vi "Launcher - Graph Master.vi"(6 "Worker Alias":string="Graph Master", 8 "error in":errorcluster, 9 "Initialization Data":T1, 11 "Graph Master in":refnum<class "Graph Master.lvclass">) -> (0 "error out":errorcluster)   [LabVIEW 2023, in "Graph Master.lvclass"]
doc: "This VI launches the Head Worker of a Workers application."
uses:
  Graph Master.lvclass
  Initialization Data.ctl
  Response Cases.ctl
  C:/Program Files/National Instruments/LabVIEW 2023/vi.lib/addons/_Workers/Library/Classes/Worker/Worker.lvclass
  Graph Master.lvclass/Graph Master.ctl
  <vilib>/addons/_Workers/Debugger/Debug Client/Debug Client.lvlib
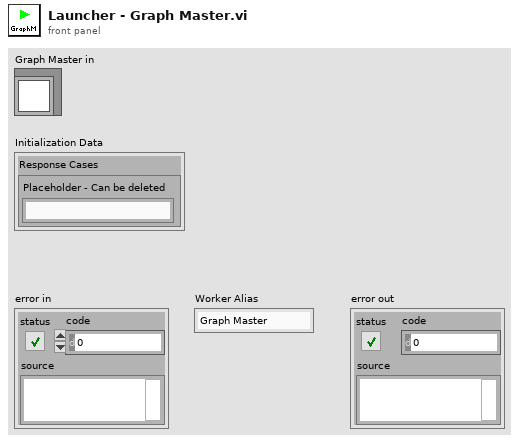
[diagram p1: front panel]
types:
  T1 = typedef "Graph Master.lvclass/Initialization Data.ctl" = cluster{"Response Cases":T2}
  T2 = typedef "Graph Master.lvclass/Response Cases.ctl" = cluster{"Placeholder - Can be deleted":string}
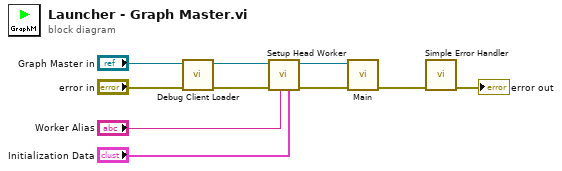
[diagram p0: block diagram]
diagram:
  n1 = call <vilib>:"Debug Client Loader.vi"("error in (no error)"="error in", "Worker_"="Graph Master in") -> ("error out"=w3:errorcluster, "Worker_out"=w1:refnum<class "Graph Master.lvclass">)  [unwired: 8 in]
  n2 = call-dynamic "Setup Head Worker.vi"("Initalization Data"="Initialization Data", "Worker Alias"="Worker Alias", "error in"=w3, "Worker_"=w1) -> ("error out"=w10:errorcluster, "Worker_out"=w7:refnum<class "Graph Master.lvclass">)  [unwired: 6 in]
  n3 = call-dynamic "Main.vi"("error in"=w10, "Graph Master in"=w7) -> ("error out"=w8:errorcluster)  [unwired: 8 in, 1 out]
  n4 = call <vilib>:"Simple Error Handler.vi"("error in (no error)"=w8) -> ("error out"=→"error out":errorcluster)  [unwired: 4 in, 4 out]
